vi "Shift ROI.vi"(8 "error in (no error)":errorcluster, 9 "Y Shift":i32, 10 "X Shift":i32, 11 "ROI":T1) -> (0 "error out":errorcluster, 3 "ROI Descriptor out":T2 {"Contours"."Type" items=["No Selection", "Point", "Line", "Rectangle", "Oval", "Polygon", "Freehand Region", "Annulus", "Unused2", "Unused3", "Broken Line", "Freehand Line", "Rotated Rectangle"]})   [LabVIEW 2023]
uses:
  <vilib>/vision/NI_Vision_Development_Module.lvlib
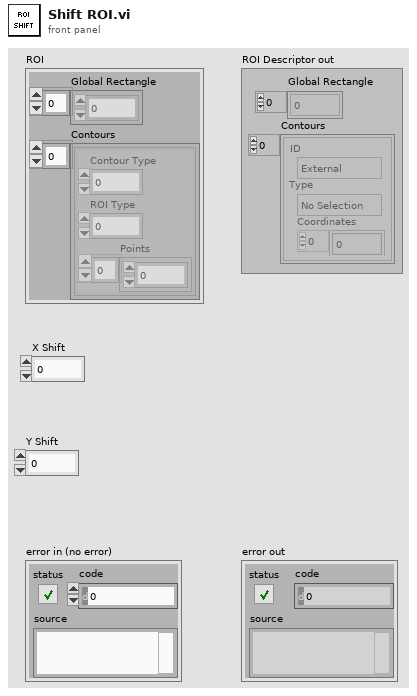
[diagram p1: front panel]
types:
  T1 = cluster{"Global Rectangle":i32[], "Contours":cluster{"Contour Type":u32, "ROI Type":u32, "Points":i32[]}[]}
  T2 = typedef "ROI Descriptor" = cluster{"Global Rectangle":i32[], "Contours":cluster{"ID":enum32{"External", "Internal"}, "Type":u32, "Coordinates":i32[]}[]}
  T3 = cluster{"Origin":cluster{"X":sgl, "Y":sgl}, "Angle (deg)":sgl, "Axis Reference":u32}
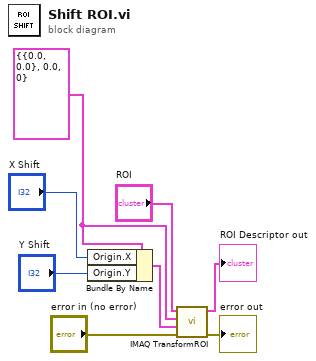
[diagram p0: block diagram]
diagram:
  w2 = T3 {"Origin"={"X"=0.0, "Y"=0.0}, "Angle (deg)"=0.0, "Axis Reference"=0} ("Base Reference")
  n1 = Bundle By Name(cluster=w2, "Origin.X"="X Shift", "Origin.Y"="Y Shift") -> (w3:T3)
  n2 = call "IMAQ TransformROI"("error in (no error)"="error in (no error)", "New Reference"=w3, "Base Reference"=w2, "ROI Descriptor"="ROI") -> ("error out"=→"error out":errorcluster, "ROI Descriptor out"=→"ROI Descriptor out":T2)  [unwired: 6 in]
